vi "new.vi"(8 "error in":errorcluster, 11 "websocket user plugin":refnum<class "websocket user plugin.lvclass">) -> (0 "error out":errorcluster, 3 "websocket upgrade handler out":refnum<class "websocket upgrade handler.lvclass">)   [LabVIEW 2016, in "websocket upgrade handler.lvclass"]
uses:
  websocket upgrade handler.lvclass
  user plugin/websocket user plugin.lvclass
  websocket upgrade handler.lvclass/websocket upgrade handler.ctl
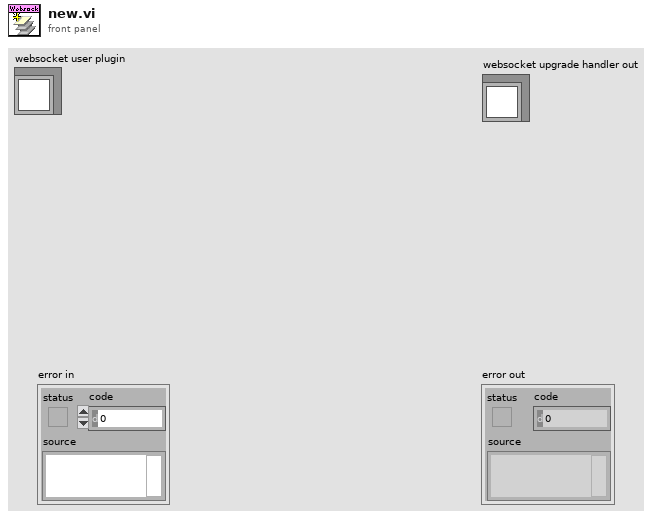
[diagram p1: front panel]
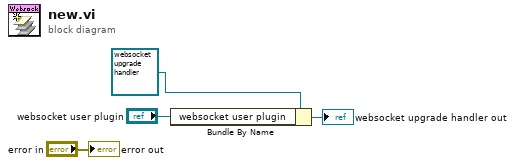
[diagram p0: block diagram]
diagram:
  n1 = Bundle By Name(cluster=refnum<class "websocket upgrade handler.lvclass"> refnum ("websocket upgrade handler in"), "websocket user plugin"="websocket user plugin") -> (→"websocket upgrade handler out":refnum<class "websocket upgrade handler.lvclass">)
  "error out" <- "error in"
